vi "final_project.vi"() -> ()   [LabVIEW 2015]
panel:
  out "Red 2":bool
  out "Yellow 2":bool
  out "Orange 2":bool
  out "Green":bool
  out "violet":bool
  out "blue":bool
  out "indigo":bool
  in  "7":bool
  out "Red 7":bool
  out "Yellow 5":bool
  out "Orange 6":bool
  out "Green 4":bool
  out "blue 3":bool
  out "indigo 2":bool
  in  "6":bool
  out "Red 6":bool
  out "Yellow 4":bool
  out "Orange 5":bool
  out "Green 3":bool
  out "blue 2":bool
  in  "5":bool
  out "Red 5":bool
  out "Yellow 3":bool
  out "Orange 4":bool
  out "Green 2":bool
  in  "4":bool
  out "Red 4":bool
  out "Orange 3":bool
  in  "2":bool
  out "Red 3":bool
  in  "1":bool
  in  "Boolean0":bool
  out "?":bool
  out "?":bool
  out "?":bool
  out "?":bool
  out "?":bool
  out "?":bool
  out "?":bool
  out "Red":bool
  out "Yellow":bool
  out "Orange":bool
  in  "3":bool
  in  "Numeric":i32
  # "This 7 seg shows the previous state as we start from 0"
  # "before run the program please make sure you put 0 in Numeric then pur the number you want to go \nexample : 3 then press stop 3 then wait for 2 seconds  ... put ur second number (for example 7) then stop 7 ...etc."
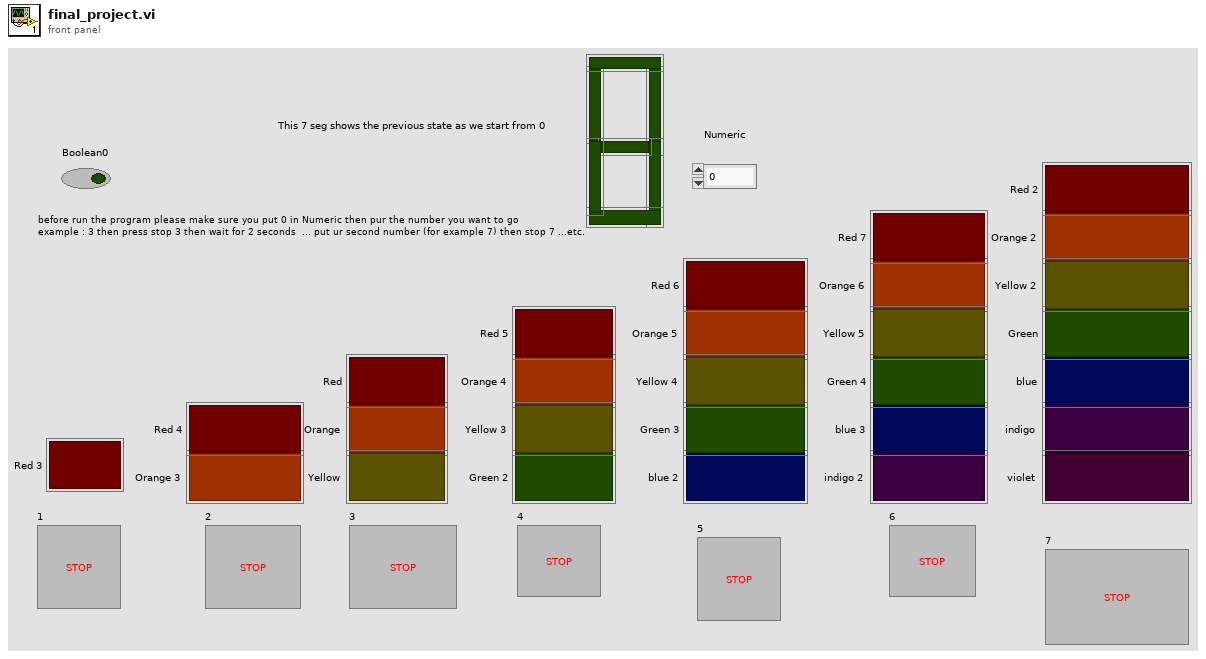
[diagram p1: front panel]
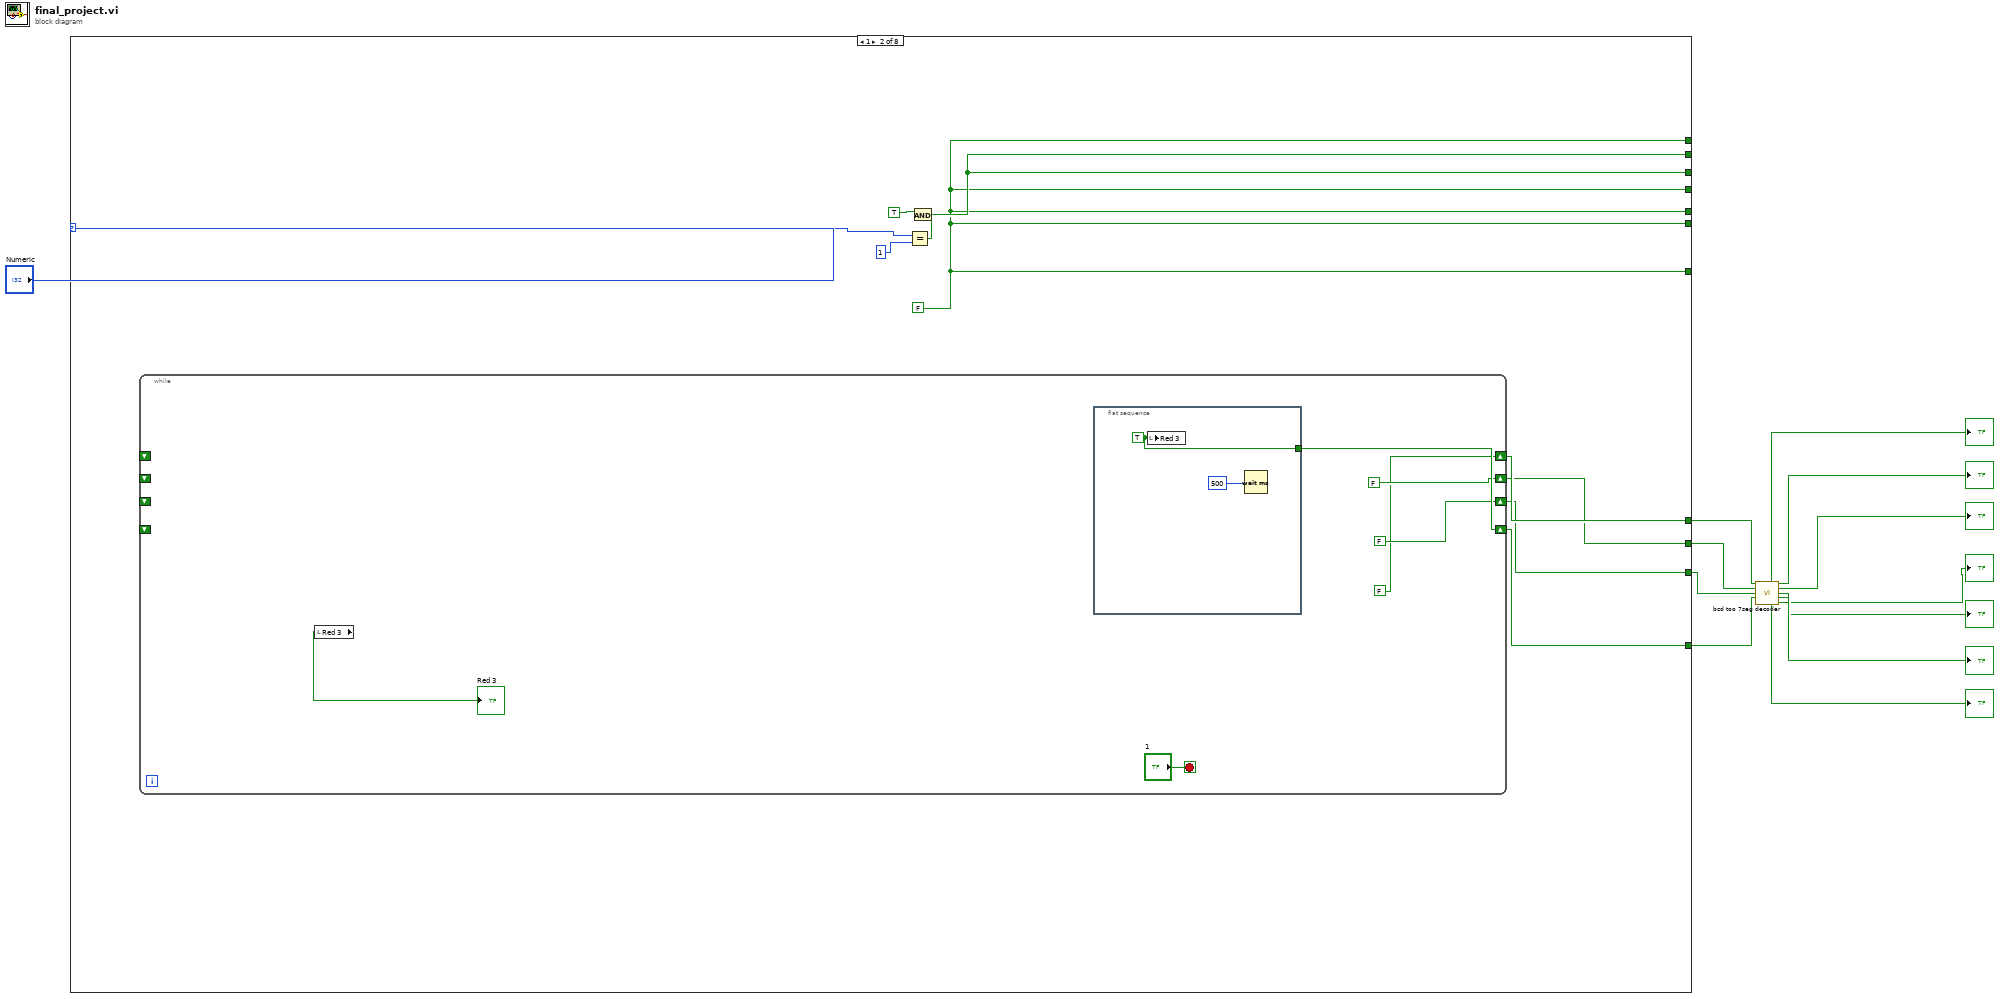
[diagram p0: block diagram]
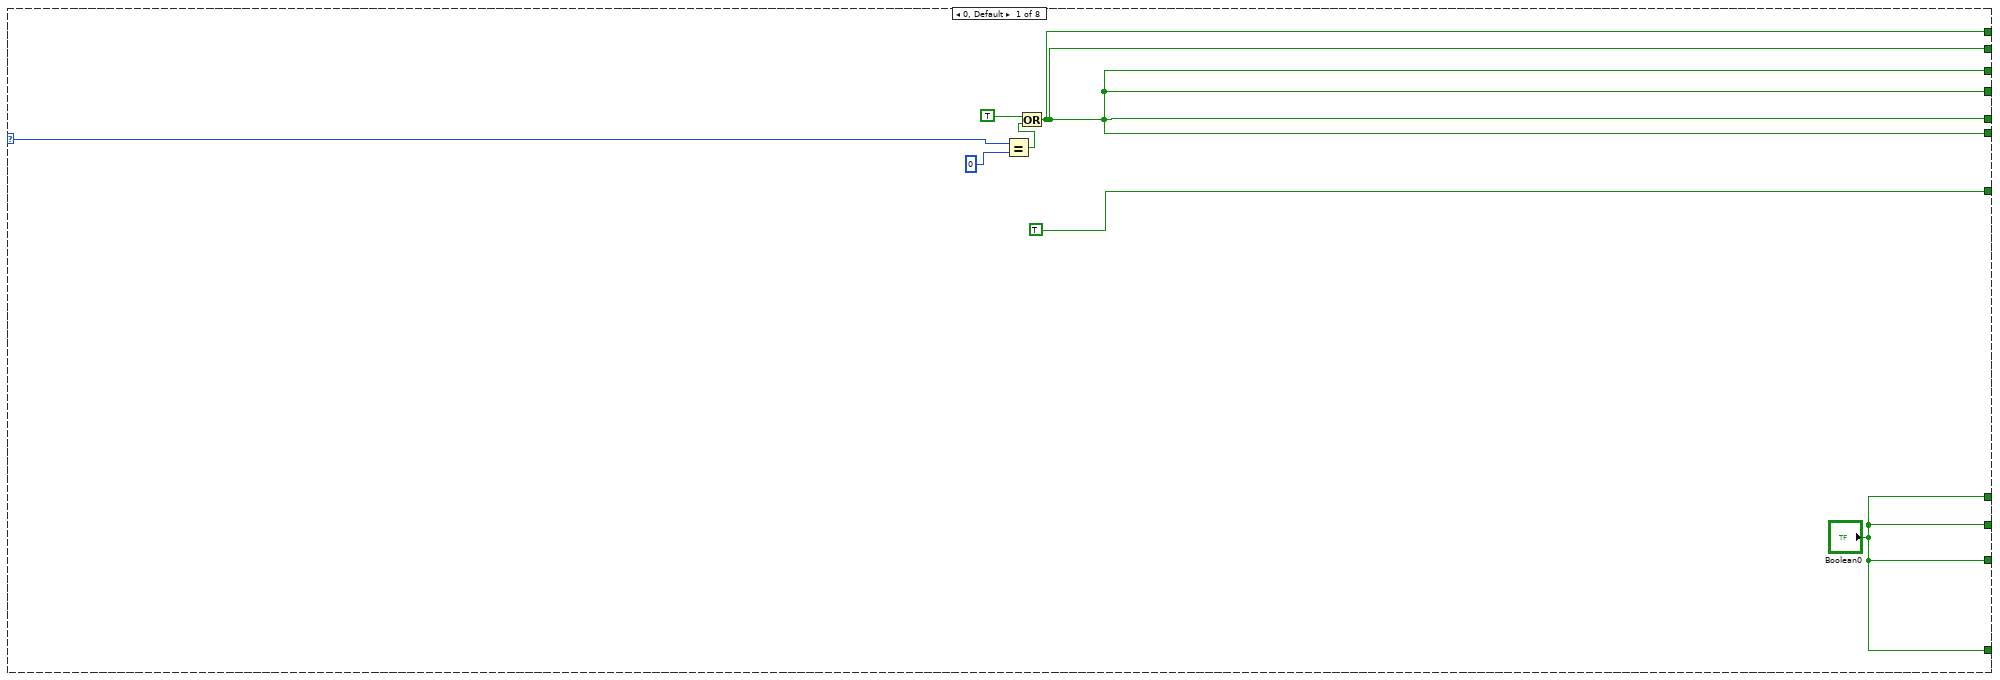
[diagram p2: hidden frame]
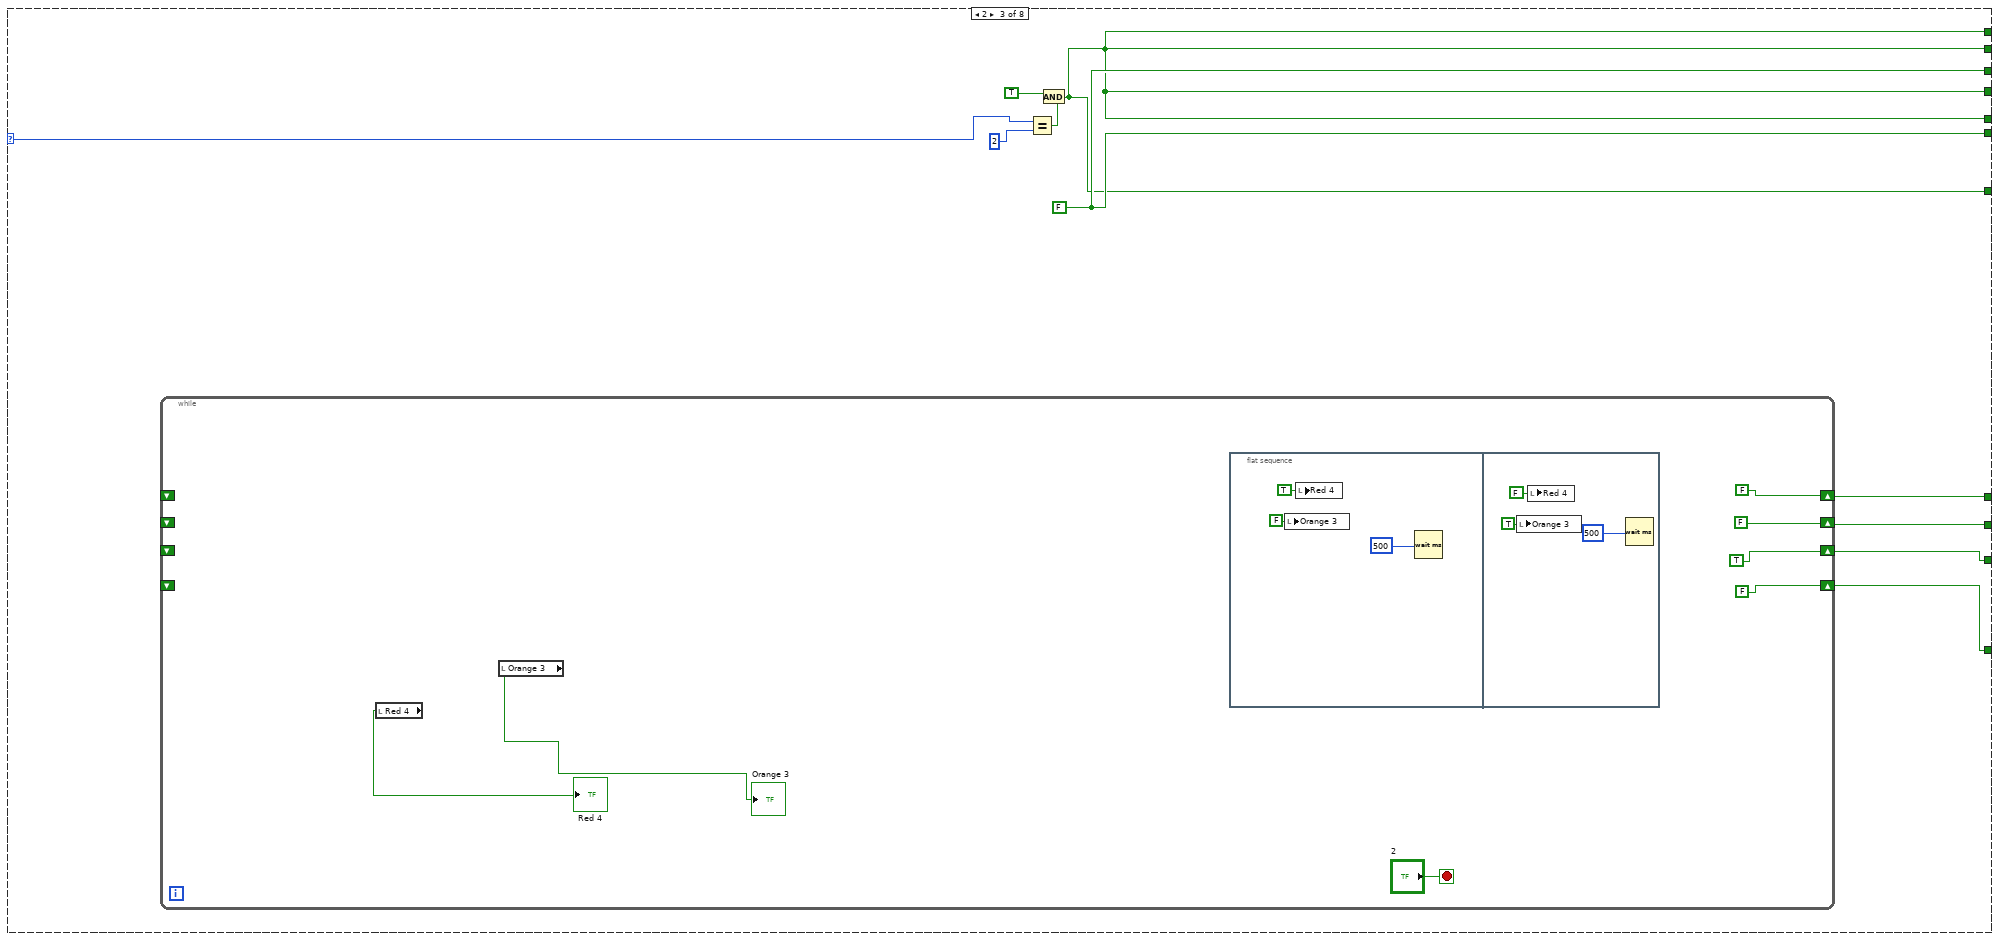
[diagram p3: hidden frame]
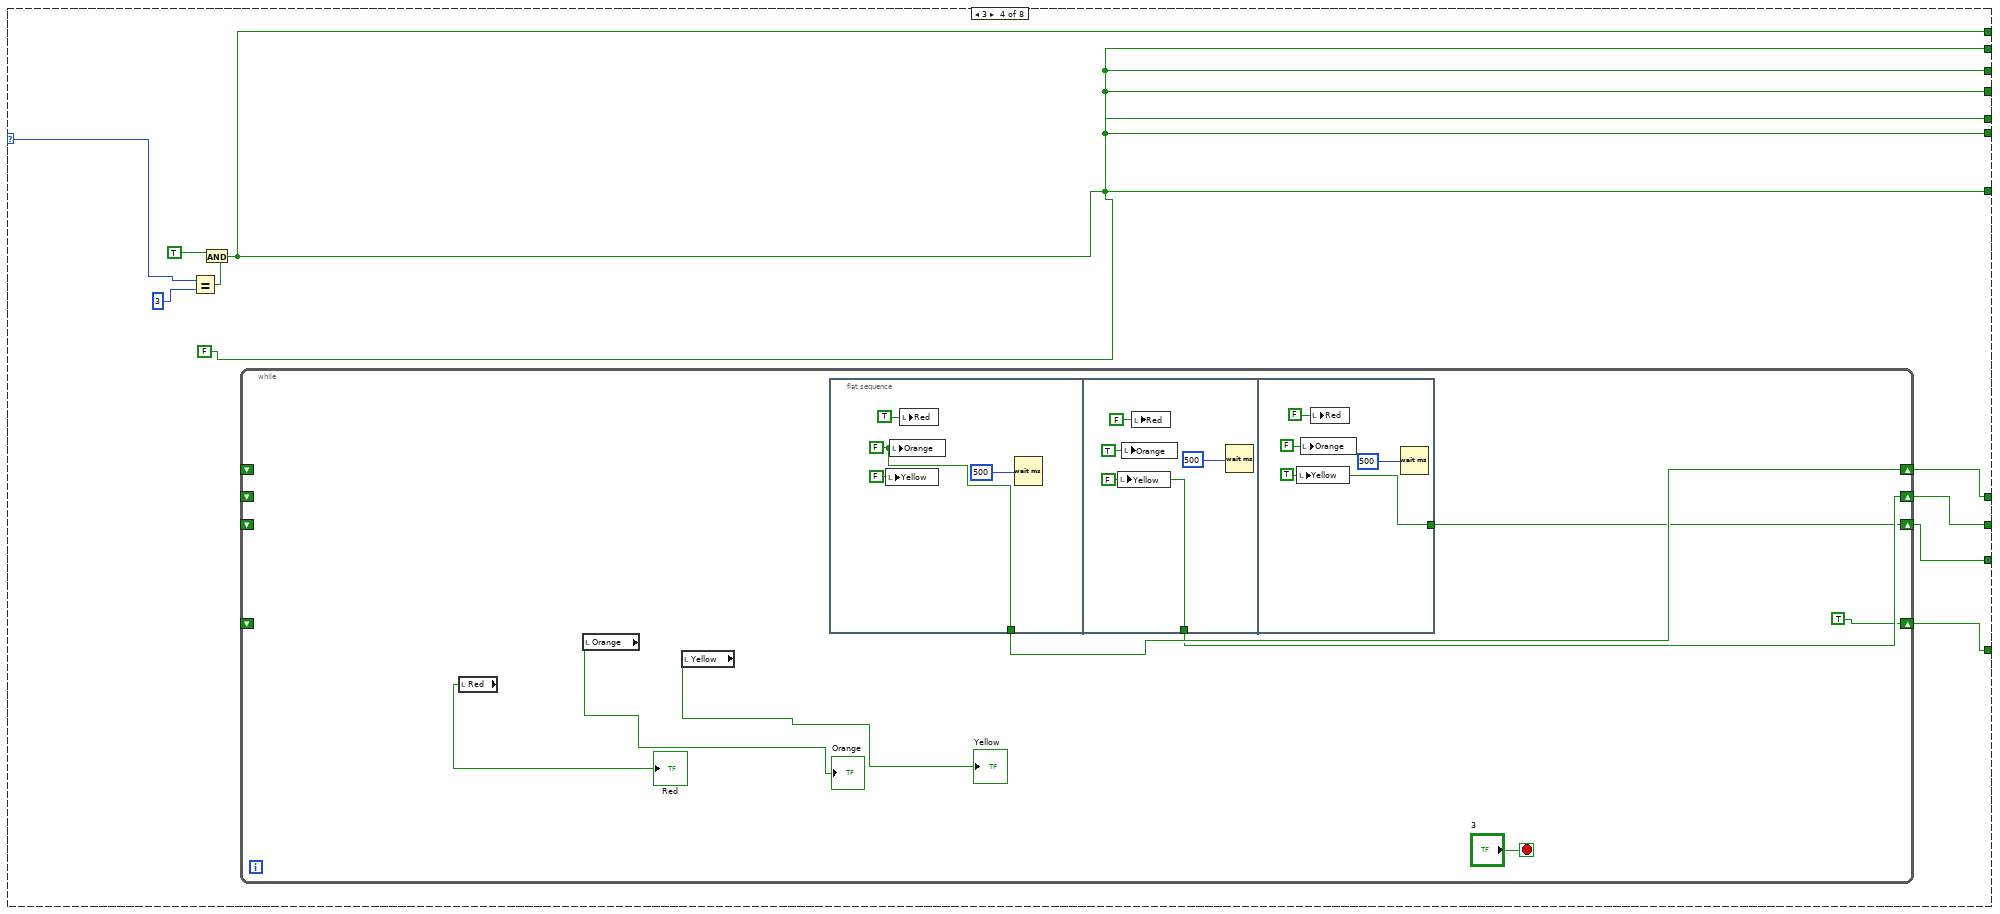
[diagram p4: hidden frame]
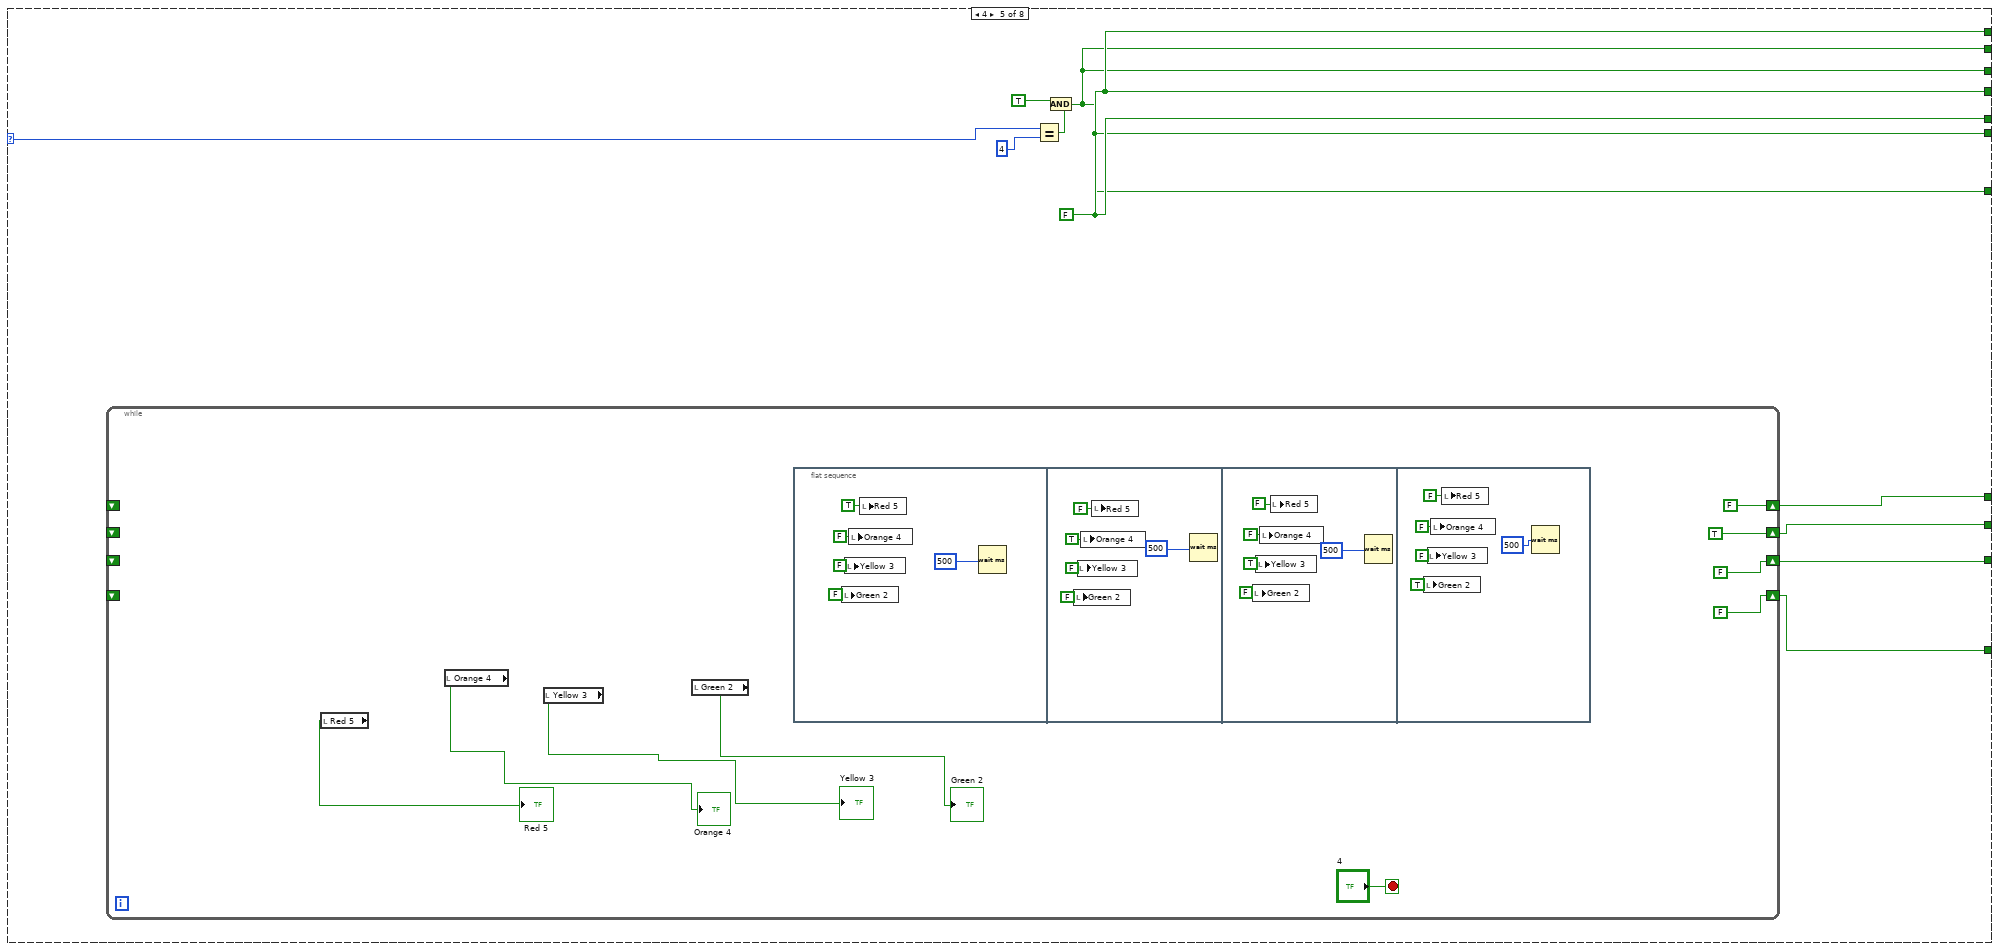
[diagram p5: hidden frame]
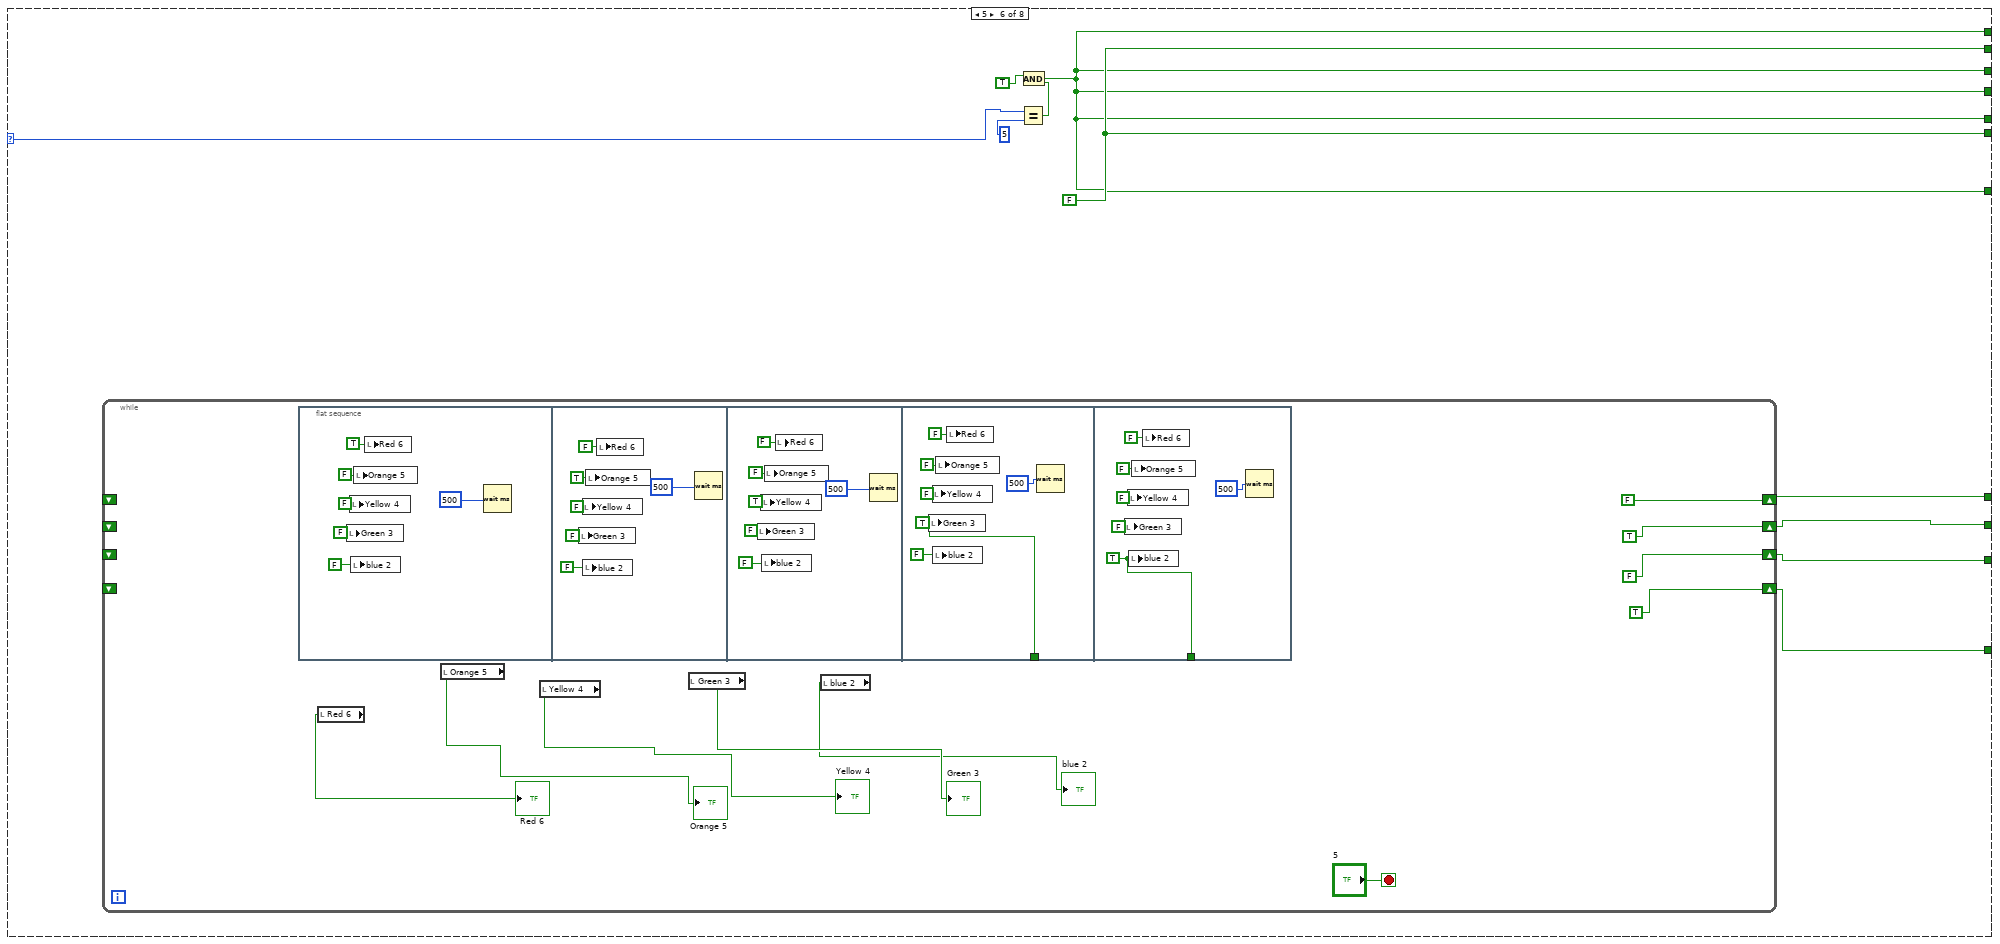
[diagram p6: hidden frame]
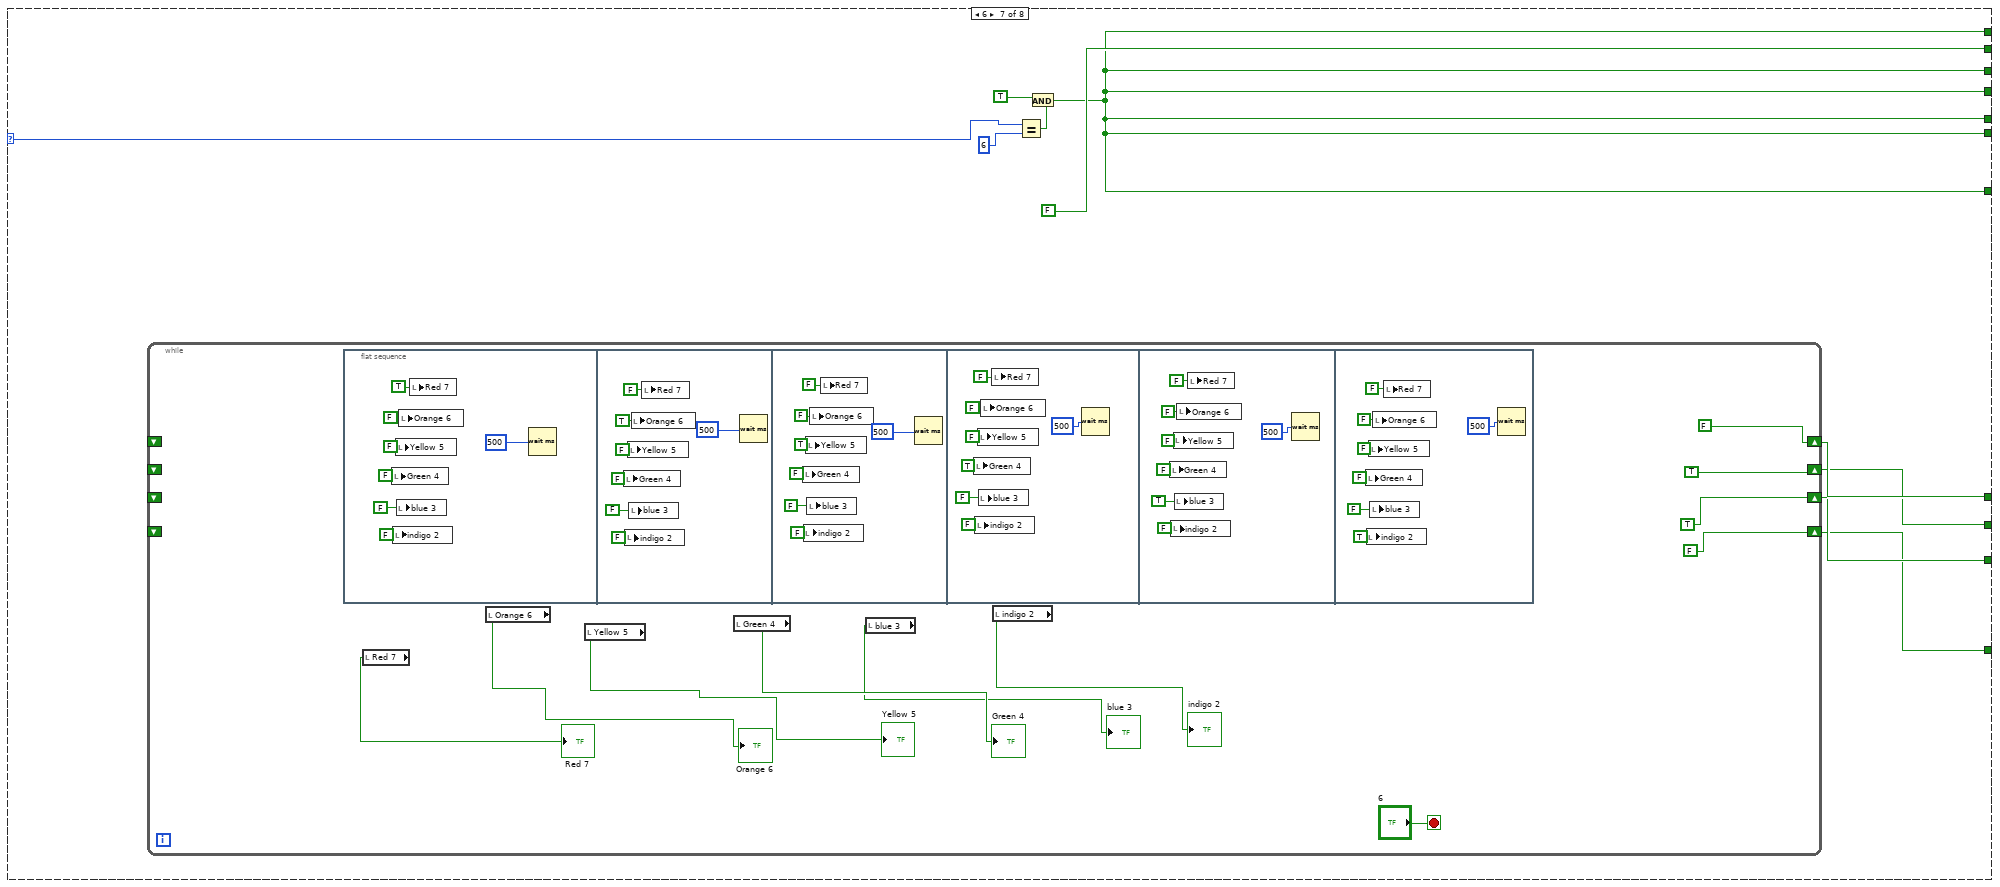
[diagram p7: hidden frame]
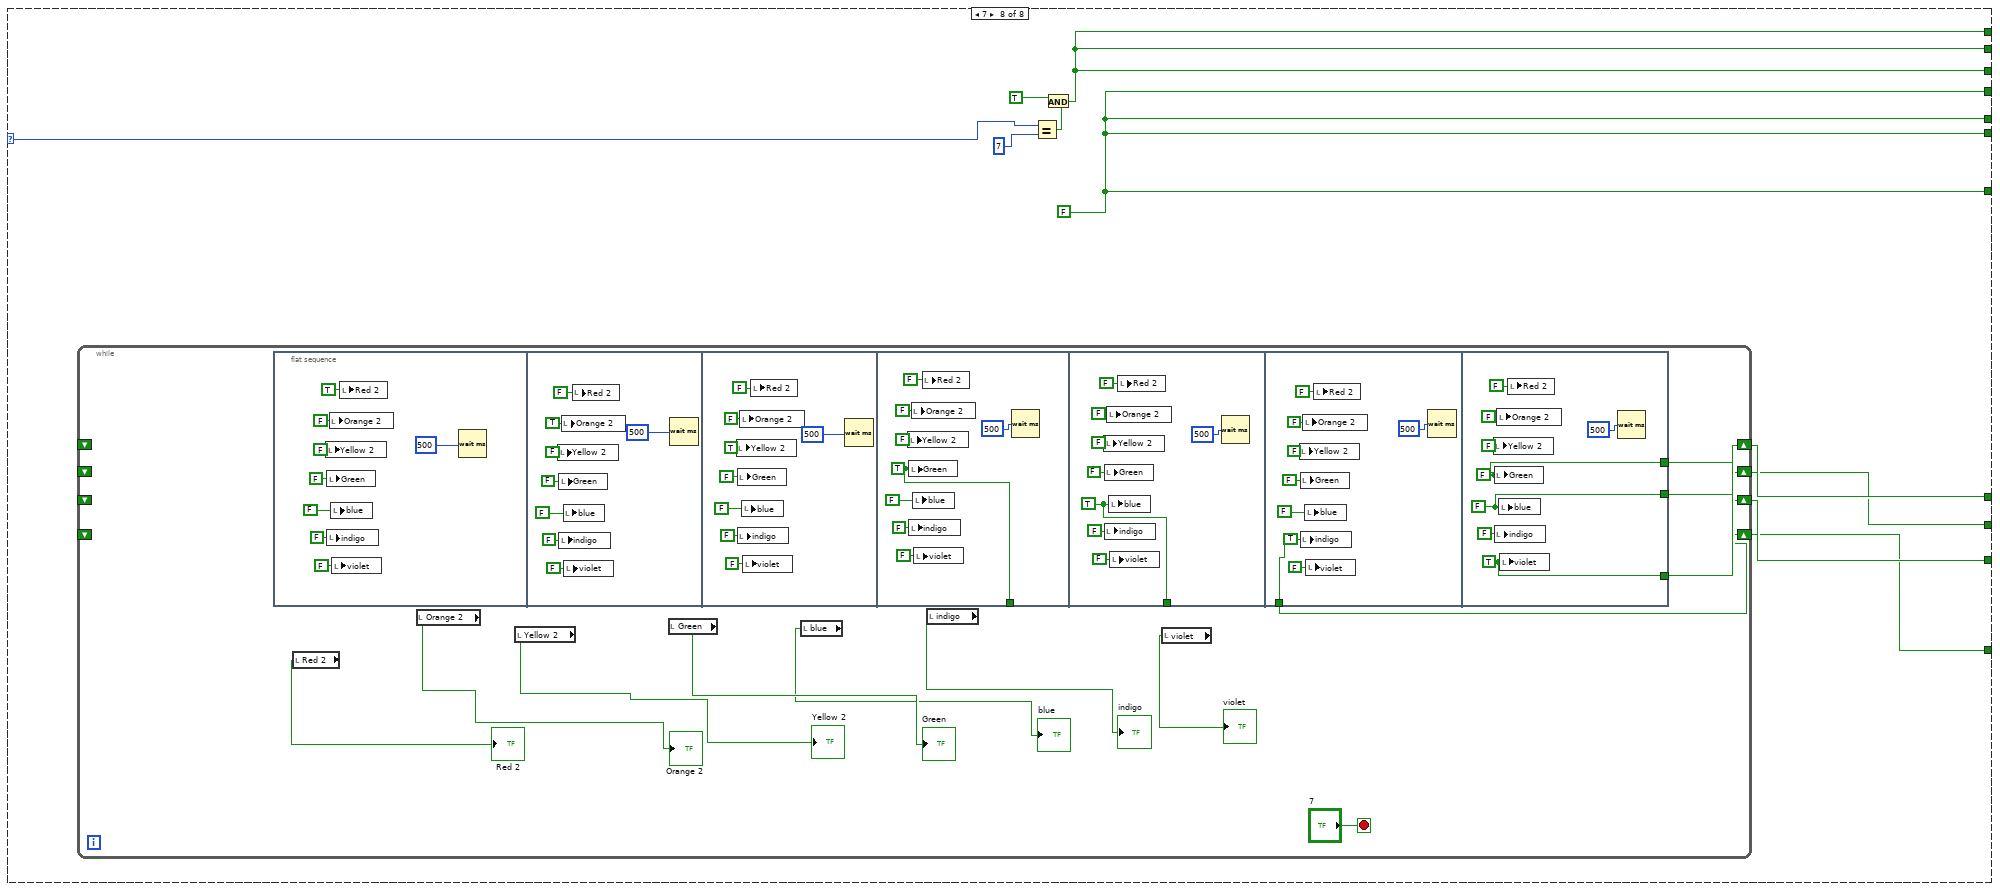
[diagram p8: hidden frame]
diagram:
  n1 = case shown="1" "Numeric" {
    selector: "Numeric" -> [w19 w26 w44 w67 w97 w136 w186 w249]
    tunnel: [w15 w24 w42 w65 w96 w134 w184 w247] -> _
    tunnel: [w15 w25 w42 w65 w95 w135 FALSE w247] -> _
    tunnel: [w15 w25 w43 w65 w95 w134 w184 w247] -> _
    tunnel: [w15 w24 w42 w65 w96 w134 w184 w248] -> _
    tunnel: [w15 w24 w42 w66 w96 w134 w184 w248] -> _
    tunnel: [w15 w24 w43 w66 w95 w135 w184 w248] -> _
    tunnel: [TRUE w24 w42 w65 w95 w134 w184 w248] -> _
    tunnel: ["Boolean0" w20 w39 w62 w92 w131 w181 w244] -> w2
    tunnel: ["Boolean0" w22 w41 w64 w94 w133 w183 w246] -> w4
    tunnel: ["Boolean0" w21 w40 w63 w93 w132 w182 w245] -> w3
    tunnel: ["Boolean0" w23 w38 w61 w91 w130 w180 w243] -> w1
    frame 0, Default {
      n2 = Equal?(x=w19, y=i16 0) -> (x = y?=w16:bool)
      n3 = Or(x=TRUE, y=w16) -> (x .or. y?=w15:bool)
    }
    frame 1 {
      w24 = FALSE
      n4 = while {
        shift-right: [FALSE ("Red")] -> w22
        shift-left: _ -> [_]
        shift-right: [FALSE ("Red")] -> w21
        shift-left: _ -> [_]
        shift-right: [FALSE ("Red")] -> w20
        shift-left: _ -> [_]
        shift-right: [w33] -> w23
        shift-left: _ -> [_]
        stop <- "1" stop-if-true
        n5 = local read "Red 3"() -> (→"Red 3":bool)
        n6 = flat-sequence {
          tunnel: [w36] -> w33
          frame #0 {
            w36 = TRUE ("Red")
            n7 = local write "Red 3"(w36) -> ()
            n8 = Wait (ms)(milliseconds to wait=u32 500 ("millisecond timer value")) -> ()  [unwired: 1 out]
          }
        }
      }
      n9 = Equal?(x=w26, y=i16 1) -> (x = y?=w28:bool)
      n10 = And(x=TRUE, y=w28) -> (x .and. y?=w25:bool)
    }
    frame 2 {
      w43 = FALSE
      n11 = while {
        shift-right: [FALSE ("Red")] -> w41
        shift-left: _ -> [_]
        shift-right: [FALSE ("Red")] -> w40
        shift-left: _ -> [_]
        shift-right: [TRUE ("Red")] -> w39
        shift-left: _ -> [_]
        shift-right: [FALSE ("Red")] -> w38
        shift-left: _ -> [_]
        stop <- "2" stop-if-true
        n12 = local read "Red 4"() -> (→"Red 4":bool)
        n13 = local read "Orange 3"() -> (→"Orange 3":bool)
        n14 = flat-sequence {
          frame #0 {
            n15 = local write "Orange 3"(FALSE ("Yellow")) -> ()
            n16 = local write "Red 4"(TRUE ("Red")) -> ()
            n17 = Wait (ms)(milliseconds to wait=u32 500 ("millisecond timer value")) -> ()  [unwired: 1 out]
          }
          frame #1 {
            n18 = local write "Orange 3"(TRUE ("Yellow")) -> ()
            n19 = local write "Red 4"(FALSE ("Red")) -> ()
            n20 = Wait (ms)(milliseconds to wait=u32 500 ("millisecond timer value")) -> ()  [unwired: 1 out]
          }
        }
      }
      n21 = Equal?(x=w44, y=i16 2) -> (x = y?=w46:bool)
      n22 = And(x=TRUE, y=w46) -> (x .and. y?=w42:bool)
    }
    frame 3 {
      w66 = FALSE
      n23 = Equal?(x=w67, y=i16 3) -> (x = y?=w69:bool)
      n24 = And(x=TRUE, y=w69) -> (x .and. y?=w65:bool)
      n25 = while {
        shift-right: [w74] -> w64
        shift-left: _ -> [_]
        shift-right: [w73] -> w63
        shift-left: _ -> [_]
        shift-right: [w72] -> w62
        shift-left: _ -> [_]
        shift-right: [TRUE ("Blue")] -> w61
        shift-left: _ -> [_]
        stop <- "3" stop-if-true
        n26 = local read "Red"() -> (→"Red":bool)
        n27 = local read "Orange"() -> (→"Orange":bool)
        n28 = local read "Yellow"() -> (→"Yellow":bool)
        n29 = flat-sequence {
          tunnel: [w79] -> w74
          tunnel: [w83] -> w73
          tunnel: [w87] -> w72
          frame #0 {
            w79 = FALSE ("Yellow")
            n30 = local write "Yellow"(FALSE ("Blue")) -> ()
            n31 = local write "Orange"(w79) -> ()
            n32 = local write "Red"(TRUE ("Red")) -> ()
            n33 = Wait (ms)(milliseconds to wait=u32 500 ("millisecond timer value")) -> ()  [unwired: 1 out]
          }
          frame #1 {
            w83 = FALSE ("Blue")
            n34 = local write "Yellow"(w83) -> ()
            n35 = local write "Orange"(TRUE ("Yellow")) -> ()
            n36 = local write "Red"(FALSE ("Red")) -> ()
            n37 = Wait (ms)(milliseconds to wait=u32 500 ("millisecond timer value")) -> ()  [unwired: 1 out]
          }
          frame #2 {
            w87 = TRUE ("Blue")
            n38 = local write "Yellow"(w87) -> ()
            n39 = local write "Orange"(FALSE ("Yellow")) -> ()
            n40 = local write "Red"(FALSE ("Red")) -> ()
            n41 = Wait (ms)(milliseconds to wait=u32 500 ("millisecond timer value")) -> ()  [unwired: 1 out]
          }
        }
      }
    }
    frame 4 {
      w96 = FALSE
      n42 = while {
        shift-right: [FALSE ("Red")] -> w94
        shift-left: _ -> [_]
        shift-right: [TRUE ("Red")] -> w93
        shift-left: _ -> [_]
        shift-right: [FALSE ("Red")] -> w92
        shift-left: _ -> [_]
        shift-right: [FALSE ("Red")] -> w91
        shift-left: _ -> [_]
        stop <- "4" stop-if-true
        n43 = local read "Red 5"() -> (→"Red 5":bool)
        n44 = local read "Orange 4"() -> (→"Orange 4":bool)
        n45 = local read "Yellow 3"() -> (→"Yellow 3":bool)
        n46 = local read "Green 2"() -> (→"Green 2":bool)
        n47 = flat-sequence {
          frame #0 {
            n48 = local write "Green 2"(FALSE ("Red")) -> ()
            n49 = local write "Yellow 3"(FALSE ("Blue")) -> ()
            n50 = local write "Orange 4"(FALSE ("Yellow")) -> ()
            n51 = local write "Red 5"(TRUE ("Red")) -> ()
            n52 = Wait (ms)(milliseconds to wait=u32 500 ("millisecond timer value")) -> ()  [unwired: 1 out]
          }
          frame #1 {
            n53 = local write "Green 2"(FALSE ("Red")) -> ()
            n54 = local write "Yellow 3"(FALSE ("Blue")) -> ()
            n55 = local write "Orange 4"(TRUE ("Yellow")) -> ()
            n56 = local write "Red 5"(FALSE ("Red")) -> ()
            n57 = Wait (ms)(milliseconds to wait=u32 500 ("millisecond timer value")) -> ()  [unwired: 1 out]
          }
          frame #2 {
            n58 = local write "Green 2"(FALSE ("Red")) -> ()
            n59 = local write "Yellow 3"(TRUE ("Blue")) -> ()
            n60 = local write "Orange 4"(FALSE ("Yellow")) -> ()
            n61 = local write "Red 5"(FALSE ("Red")) -> ()
            n62 = Wait (ms)(milliseconds to wait=u32 500 ("millisecond timer value")) -> ()  [unwired: 1 out]
          }
          frame #3 {
            n63 = local write "Green 2"(TRUE ("Red")) -> ()
            n64 = local write "Yellow 3"(FALSE ("Blue")) -> ()
            n65 = local write "Orange 4"(FALSE ("Yellow")) -> ()
            n66 = local write "Red 5"(FALSE ("Red")) -> ()
            n67 = Wait (ms)(milliseconds to wait=u32 500 ("millisecond timer value")) -> ()  [unwired: 1 out]
          }
        }
      }
      n68 = Equal?(x=w97, y=i16 4) -> (x = y?=w99:bool)
      n69 = And(x=TRUE, y=w99) -> (x .and. y?=w95:bool)
    }
    frame 5 {
      w135 = FALSE
      n70 = while {
        shift-right: [FALSE ("Red")] -> w133
        shift-left: _ -> [_]
        shift-right: [TRUE ("Red")] -> w132
        shift-left: _ -> [_]
        shift-right: [FALSE ("Red")] -> w131
        shift-left: _ -> [_]
        shift-right: [TRUE ("Red")] -> w130
        shift-left: _ -> [_]
        stop <- "5" stop-if-true
        n71 = flat-sequence {
          tunnel: [w168] -> _
          tunnel: [w174] -> _
          frame #0 {
            n72 = local write "Green 3"(FALSE ("Red")) -> ()
            n73 = local write "Yellow 4"(FALSE ("Blue")) -> ()
            n74 = local write "blue 2"(FALSE ("Yellow")) -> ()
            n75 = local write "Orange 5"(FALSE ("Yellow")) -> ()
            n76 = local write "Red 6"(TRUE ("Red")) -> ()
            n77 = Wait (ms)(milliseconds to wait=u32 500 ("millisecond timer value")) -> ()  [unwired: 1 out]
          }
          frame #1 {
            n78 = local write "Green 3"(FALSE ("Red")) -> ()
            n79 = local write "Yellow 4"(FALSE ("Blue")) -> ()
            n80 = local write "blue 2"(FALSE ("Yellow")) -> ()
            n81 = local write "Orange 5"(TRUE ("Yellow")) -> ()
            n82 = local write "Red 6"(FALSE ("Red")) -> ()
            n83 = Wait (ms)(milliseconds to wait=u32 500 ("millisecond timer value")) -> ()  [unwired: 1 out]
          }
          frame #2 {
            n84 = local write "Green 3"(FALSE ("Red")) -> ()
            n85 = local write "Yellow 4"(TRUE ("Blue")) -> ()
            n86 = local write "blue 2"(FALSE ("Yellow")) -> ()
            n87 = local write "Orange 5"(FALSE ("Yellow")) -> ()
            n88 = local write "Red 6"(FALSE ("Red")) -> ()
            n89 = Wait (ms)(milliseconds to wait=u32 500 ("millisecond timer value")) -> ()  [unwired: 1 out]
          }
          frame #3 {
            w168 = TRUE ("Red")
            n90 = local write "Green 3"(w168) -> ()
            n91 = local write "Yellow 4"(FALSE ("Blue")) -> ()
            n92 = local write "blue 2"(FALSE ("Yellow")) -> ()
            n93 = local write "Orange 5"(FALSE ("Yellow")) -> ()
            n94 = local write "Red 6"(FALSE ("Red")) -> ()
            n95 = Wait (ms)(milliseconds to wait=u32 500 ("millisecond timer value")) -> ()  [unwired: 1 out]
          }
          frame #4 {
            w174 = TRUE ("Yellow")
            n96 = local write "Green 3"(FALSE ("Red")) -> ()
            n97 = local write "Yellow 4"(FALSE ("Blue")) -> ()
            n98 = local write "blue 2"(w174) -> ()
            n99 = local write "Orange 5"(FALSE ("Yellow")) -> ()
            n100 = local write "Red 6"(FALSE ("Red")) -> ()
            n101 = Wait (ms)(milliseconds to wait=u32 500 ("millisecond timer value")) -> ()  [unwired: 1 out]
          }
        }
        n102 = local read "Red 6"() -> (→"Red 6":bool)
        n103 = local read "Orange 5"() -> (→"Orange 5":bool)
        n104 = local read "Yellow 4"() -> (→"Yellow 4":bool)
        n105 = local read "Green 3"() -> (→"Green 3":bool)
        n106 = local read "blue 2"() -> (→"blue 2":bool)
      }
      n107 = Equal?(x=w136, y=i16 5) -> (x = y?=w138:bool)
      n108 = And(x=TRUE, y=w138) -> (x .and. y?=w134:bool)
    }
    frame 6 {
      n109 = while {
        shift-right: [FALSE ("Red")] -> w183
        shift-left: _ -> [_]
        shift-right: [TRUE ("Red")] -> w182
        shift-left: _ -> [_]
        shift-right: [TRUE ("Red")] -> w181
        shift-left: _ -> [_]
        shift-right: [FALSE ("Red")] -> w180
        shift-left: _ -> [_]
        stop <- "6" stop-if-true
        n110 = flat-sequence {
          frame #0 {
            n111 = local write "Green 4"(FALSE ("Red")) -> ()
            n112 = local write "indigo 2"(FALSE ("Blue")) -> ()
            n113 = local write "Yellow 5"(FALSE ("Blue")) -> ()
            n114 = local write "blue 3"(FALSE ("Yellow")) -> ()
            n115 = local write "Orange 6"(FALSE ("Yellow")) -> ()
            n116 = local write "Red 7"(TRUE ("Red")) -> ()
            n117 = Wait (ms)(milliseconds to wait=u32 500 ("millisecond timer value")) -> ()  [unwired: 1 out]
          }
          frame #1 {
            n118 = local write "Green 4"(FALSE ("Red")) -> ()
            n119 = local write "indigo 2"(FALSE ("Blue")) -> ()
            n120 = local write "Yellow 5"(FALSE ("Blue")) -> ()
            n121 = local write "blue 3"(FALSE ("Yellow")) -> ()
            n122 = local write "Orange 6"(TRUE ("Yellow")) -> ()
            n123 = local write "Red 7"(FALSE ("Red")) -> ()
            n124 = Wait (ms)(milliseconds to wait=u32 500 ("millisecond timer value")) -> ()  [unwired: 1 out]
          }
          frame #2 {
            n125 = local write "Green 4"(FALSE ("Red")) -> ()
            n126 = local write "indigo 2"(FALSE ("Blue")) -> ()
            n127 = local write "Yellow 5"(TRUE ("Blue")) -> ()
            n128 = local write "blue 3"(FALSE ("Yellow")) -> ()
            n129 = local write "Orange 6"(FALSE ("Yellow")) -> ()
            n130 = local write "Red 7"(FALSE ("Red")) -> ()
            n131 = Wait (ms)(milliseconds to wait=u32 500 ("millisecond timer value")) -> ()  [unwired: 1 out]
          }
          frame #3 {
            n132 = local write "Green 4"(TRUE ("Red")) -> ()
            n133 = local write "indigo 2"(FALSE ("Blue")) -> ()
            n134 = local write "Yellow 5"(FALSE ("Blue")) -> ()
            n135 = local write "blue 3"(FALSE ("Yellow")) -> ()
            n136 = local write "Orange 6"(FALSE ("Yellow")) -> ()
            n137 = local write "Red 7"(FALSE ("Red")) -> ()
            n138 = Wait (ms)(milliseconds to wait=u32 500 ("millisecond timer value")) -> ()  [unwired: 1 out]
          }
          frame #4 {
            n139 = local write "Green 4"(FALSE ("Red")) -> ()
            n140 = local write "indigo 2"(FALSE ("Blue")) -> ()
            n141 = local write "Yellow 5"(FALSE ("Blue")) -> ()
            n142 = local write "blue 3"(TRUE ("Yellow")) -> ()
            n143 = local write "Orange 6"(FALSE ("Yellow")) -> ()
            n144 = local write "Red 7"(FALSE ("Red")) -> ()
            n145 = Wait (ms)(milliseconds to wait=u32 500 ("millisecond timer value")) -> ()  [unwired: 1 out]
          }
          frame #5 {
            n146 = local write "Green 4"(FALSE ("Red")) -> ()
            n147 = local write "indigo 2"(TRUE ("Blue")) -> ()
            n148 = local write "Yellow 5"(FALSE ("Blue")) -> ()
            n149 = local write "blue 3"(FALSE ("Yellow")) -> ()
            n150 = local write "Orange 6"(FALSE ("Yellow")) -> ()
            n151 = local write "Red 7"(FALSE ("Red")) -> ()
            n152 = Wait (ms)(milliseconds to wait=u32 500 ("millisecond timer value")) -> ()  [unwired: 1 out]
          }
        }
        n153 = local read "Red 7"() -> (→"Red 7":bool)
        n154 = local read "Orange 6"() -> (→"Orange 6":bool)
        n155 = local read "Yellow 5"() -> (→"Yellow 5":bool)
        n156 = local read "Green 4"() -> (→"Green 4":bool)
        n157 = local read "blue 3"() -> (→"blue 3":bool)
        n158 = local read "indigo 2"() -> (→"indigo 2":bool)
      }
      n159 = Equal?(x=w186, y=i16 6) -> (x = y?=w188:bool)
      n160 = And(x=TRUE, y=w188) -> (x .and. y?=w184:bool)
    }
    frame 7 {
      w248 = FALSE
      n161 = while {
        shift-right: [w256] -> w246
        shift-left: _ -> [_]
        shift-right: [w255] -> w245
        shift-left: _ -> [_]
        shift-right: [w254] -> w244
        shift-left: _ -> [_]
        shift-right: [w253] -> w243
        shift-left: _ -> [_]
        stop <- "7" stop-if-true
        n162 = flat-sequence {
          tunnel: [w289] -> _
          tunnel: [w297] -> _
          tunnel: [w306] -> w253
          tunnel: [w315] -> w256
          tunnel: [w314] -> w255
          tunnel: [w313] -> w254
          frame #0 {
            n163 = local write "Yellow 2"(FALSE ("Blue")) -> ()
            n164 = local write "Green"(FALSE ("Red")) -> ()
            n165 = local write "indigo"(FALSE ("Blue")) -> ()
            n166 = local write "Orange 2"(FALSE ("Yellow")) -> ()
            n167 = local write "blue"(FALSE ("Yellow")) -> ()
            n168 = local write "violet"(FALSE ("Blue")) -> ()
            n169 = local write "Red 2"(TRUE ("Red")) -> ()
            n170 = Wait (ms)(milliseconds to wait=u32 500 ("millisecond timer value")) -> ()  [unwired: 1 out]
          }
          frame #1 {
            n171 = local write "Yellow 2"(FALSE ("Blue")) -> ()
            n172 = local write "Green"(FALSE ("Red")) -> ()
            n173 = local write "indigo"(FALSE ("Blue")) -> ()
            n174 = local write "Orange 2"(TRUE ("Yellow")) -> ()
            n175 = local write "blue"(FALSE ("Yellow")) -> ()
            n176 = local write "violet"(FALSE ("Blue")) -> ()
            n177 = local write "Red 2"(FALSE ("Red")) -> ()
            n178 = Wait (ms)(milliseconds to wait=u32 500 ("millisecond timer value")) -> ()  [unwired: 1 out]
          }
          frame #2 {
            n179 = local write "Yellow 2"(TRUE ("Blue")) -> ()
            n180 = local write "Green"(FALSE ("Red")) -> ()
            n181 = local write "indigo"(FALSE ("Blue")) -> ()
            n182 = local write "Orange 2"(FALSE ("Yellow")) -> ()
            n183 = local write "blue"(FALSE ("Yellow")) -> ()
            n184 = local write "violet"(FALSE ("Blue")) -> ()
            n185 = local write "Red 2"(FALSE ("Red")) -> ()
            n186 = Wait (ms)(milliseconds to wait=u32 500 ("millisecond timer value")) -> ()  [unwired: 1 out]
          }
          frame #3 {
            w289 = TRUE ("Red")
            n187 = local write "Yellow 2"(FALSE ("Blue")) -> ()
            n188 = local write "Green"(w289) -> ()
            n189 = local write "indigo"(FALSE ("Blue")) -> ()
            n190 = local write "Orange 2"(FALSE ("Yellow")) -> ()
            n191 = local write "blue"(FALSE ("Yellow")) -> ()
            n192 = local write "violet"(FALSE ("Blue")) -> ()
            n193 = local write "Red 2"(FALSE ("Red")) -> ()
            n194 = Wait (ms)(milliseconds to wait=u32 500 ("millisecond timer value")) -> ()  [unwired: 1 out]
          }
          frame #4 {
            w297 = TRUE ("Yellow")
            n195 = local write "Yellow 2"(FALSE ("Blue")) -> ()
            n196 = local write "Green"(FALSE ("Red")) -> ()
            n197 = local write "indigo"(FALSE ("Blue")) -> ()
            n198 = local write "Orange 2"(FALSE ("Yellow")) -> ()
            n199 = local write "blue"(w297) -> ()
            n200 = local write "violet"(FALSE ("Blue")) -> ()
            n201 = local write "Red 2"(FALSE ("Red")) -> ()
            n202 = Wait (ms)(milliseconds to wait=u32 500 ("millisecond timer value")) -> ()  [unwired: 1 out]
          }
          frame #5 {
            w306 = TRUE ("Blue")
            n203 = local write "Yellow 2"(FALSE ("Blue")) -> ()
            n204 = local write "Green"(FALSE ("Red")) -> ()
            n205 = local write "indigo"(w306) -> ()
            n206 = local write "Orange 2"(FALSE ("Yellow")) -> ()
            n207 = local write "blue"(FALSE ("Yellow")) -> ()
            n208 = local write "violet"(FALSE ("Blue")) -> ()
            n209 = local write "Red 2"(FALSE ("Red")) -> ()
            n210 = Wait (ms)(milliseconds to wait=u32 500 ("millisecond timer value")) -> ()  [unwired: 1 out]
          }
          frame #6 {
            w315 = TRUE ("Blue")
            w313 = FALSE ("Yellow")
            w314 = FALSE ("Red")
            n211 = local write "Yellow 2"(FALSE ("Blue")) -> ()
            n212 = local write "Green"(w314) -> ()
            n213 = local write "indigo"(FALSE ("Blue")) -> ()
            n214 = local write "Orange 2"(FALSE ("Yellow")) -> ()
            n215 = local write "blue"(w313) -> ()
            n216 = local write "violet"(w315) -> ()
            n217 = local write "Red 2"(FALSE ("Red")) -> ()
            n218 = Wait (ms)(milliseconds to wait=u32 500 ("millisecond timer value")) -> ()  [unwired: 1 out]
          }
        }
        n219 = local read "Red 2"() -> (→"Red 2":bool)
        n220 = local read "Orange 2"() -> (→"Orange 2":bool)
        n221 = local read "Yellow 2"() -> (→"Yellow 2":bool)
        n222 = local read "Green"() -> (→"Green":bool)
        n223 = local read "blue"() -> (→"blue":bool)
        n224 = local read "indigo"() -> (→"indigo":bool)
        n225 = local read "violet"() -> (→"violet":bool)
      }
      n226 = Equal?(x=w249, y=i16 7) -> (x = y?=w251:bool)
      n227 = And(x=TRUE, y=w251) -> (x .and. y?=w247:bool)
    }
  }
  n228 = call "bcd too 7seg decoder.vi"("A"=w4, "B"=w3, "C"=w2, "D"=w1) -> (3:→"?":bool, 4:→"?":bool, 6:→"?":bool, 8:→"?":bool, 10:→"?":bool, 14:→"?":bool, 15:→"?":bool)  [unwired: 5 in]
